vi "fgv_session_error_info.vi"(4 "Session Error Info in (\"\")":string caption="Session Info in", 5 "Operation":T1(ring), 7 "Session in":refnum<visa-resource-name> caption="VISA resource name") -> (0 "Session Error Info out":string caption="Session Info out")   [LabVIEW 2014, in "rszvl_rsidr_core.lvlib"]
uses:
  rszvl_rsidr_core.lvlib
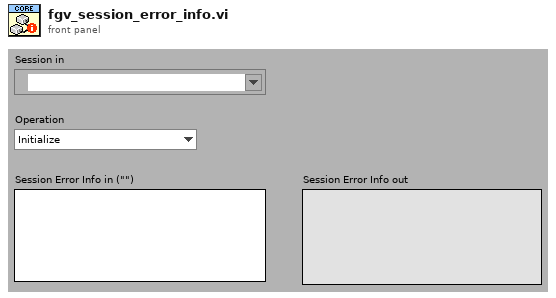
[diagram p1: front panel]
types:
  T1 = enum16{"Initialize", "GetData", "SetData", "Clear"}
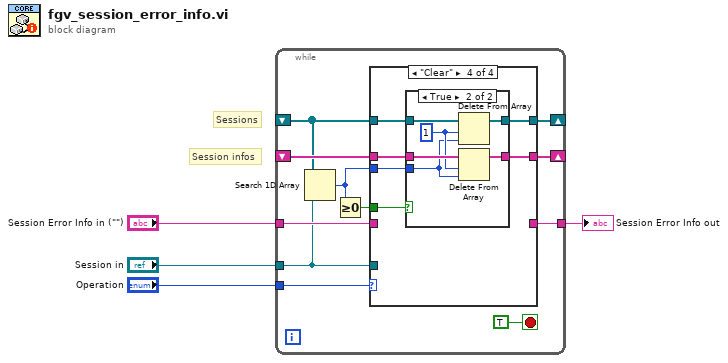
[diagram p0: block diagram]
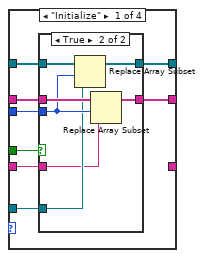
[diagram p2: hidden frame]
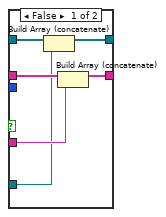
[diagram p3: hidden frame]
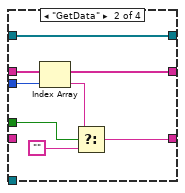
[diagram p4: hidden frame]
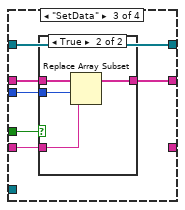
[diagram p5: hidden frame]
diagram:
  # "Session infos"
  # "Sessions"
  n1 = while {
    tunnel: [w9] -> w3
    tunnel: "Session Error Info in (\"\")" -> [w15]
    tunnel: "Operation" -> [w14]
    tunnel: "Session in" -> [w7]
    shift-right: [w13] -> _
    shift-left: _ -> [w8]
    shift-right: [w10] -> _
    shift-left: _ -> [w11]
    stop <- TRUE stop-if-true
    n2 = Search 1D Array(1D array=w8, element=w7) -> (index of element=w5:i32)  [unwired: 1 in]
    n3 = Greater Or Equal To 0?(x=w5) -> (x >= 0?=w6:bool)
    n4 = case "Operation case" shown="\"Clear\"" w14 {
      tunnel: w7 -> [w18 _ _ _]
      tunnel: w8 -> [w19 w42 w46 w58]
      tunnel: w15 -> [w22 _ w48 _]
      tunnel: [w21 w42 w46 w57] -> w13
      tunnel: w11 -> [w23 w43 w49 w60]
      tunnel: [w20 w43 w47 w59] -> w10
      tunnel: [_ w40 _ _] -> w9
      tunnel: w6 -> [w16 w37 w45 w56]
      tunnel: w5 -> [w17 w38 w44 w55]
      frame "Initialize" {
        n5 = case shown="True" w16 {
          tunnel: w23 -> [w27 w36]
          tunnel: w22 -> [w26 w30]
          tunnel: w17 -> [_ w32]
          tunnel: w18 -> [w25 w31]
          tunnel: w19 -> [w29 w34]
          tunnel: [w28 w33] -> w21
          tunnel: [w24 w35] -> w20
          frame False {
            n6 = Build Array (concatenate)(w29, w25) -> (w28:refnum<visa-resource-name>[])
            n7 = Build Array (concatenate)(w27, w26) -> (w24:string[])
          }
          frame True {
            n8 = Replace Array Subset(array=w34, new element=w31, index=w32) -> (w33:refnum<visa-resource-name>[])
            n9 = Replace Array Subset(array=w36, new element=w30, index=w32) -> (w35:string[])
          }
        }
      }
      frame "GetData" {
        n10 = Index Array(array=w43, index=w38) -> (element=w41:string)
        n11 = Select(t=w41, s=w37, f="") -> (s? t:f=w40:string)
      }
      frame "SetData" {
        n12 = case shown="True" w45 {
          tunnel: w49 -> [w50 w54]
          tunnel: w48 -> [_ w51]
          tunnel: [w50 w53] -> w47
          tunnel: w44 -> [_ w52]
          frame False {
          }
          frame True {
            n13 = Replace Array Subset(array=w54, new element=w51, index=w52) -> (w53:string[])
          }
        }
      }
      frame "Clear" {
        n14 = case shown="True" w56 {
          tunnel: w60 -> [w62 w66]
          tunnel: [w62 w65] -> w59
          tunnel: w58 -> [w61 w68]
          tunnel: [w61 w67] -> w57
          tunnel: w55 -> [_ w63]
          frame False {
          }
          frame True {
            w64 = 1 ("length")
            n15 = Delete From Array(array=w68, length=w64, index=w63) -> (array with subset deleted=w67:refnum<visa-resource-name>[])  [unwired: 1 out]
            n16 = Delete From Array(array=w66, length=w64, index=w63) -> (array with subset deleted=w65:string[])  [unwired: 1 out]
          }
        }
      }
    }
  }
  "Session Error Info out" <- w3
